vi "Open App Help file.vi"(7 "Help Tag (\"\")":string, 11 "error In":errorcluster, 13 "file name(\"App\".chm)":string) -> (15 "error out":errorcluster)   [LabVIEW 2011]
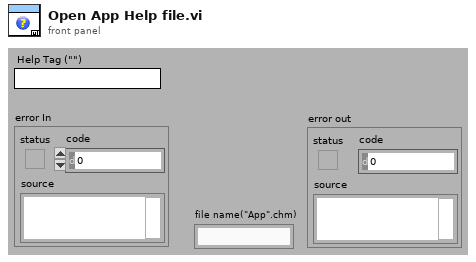
[diagram p1: front panel]
types:
  T1 = typedef "emi_Version Info.ctl" = cluster{"Name":string, "Major":i16, "Minor":i16, "Fix":i16, "Build":i32, "Type":enum16{"Alfa", "Beta", "Stable"}, "Dev":bool, "Version Name":string, "Date":timestamp}
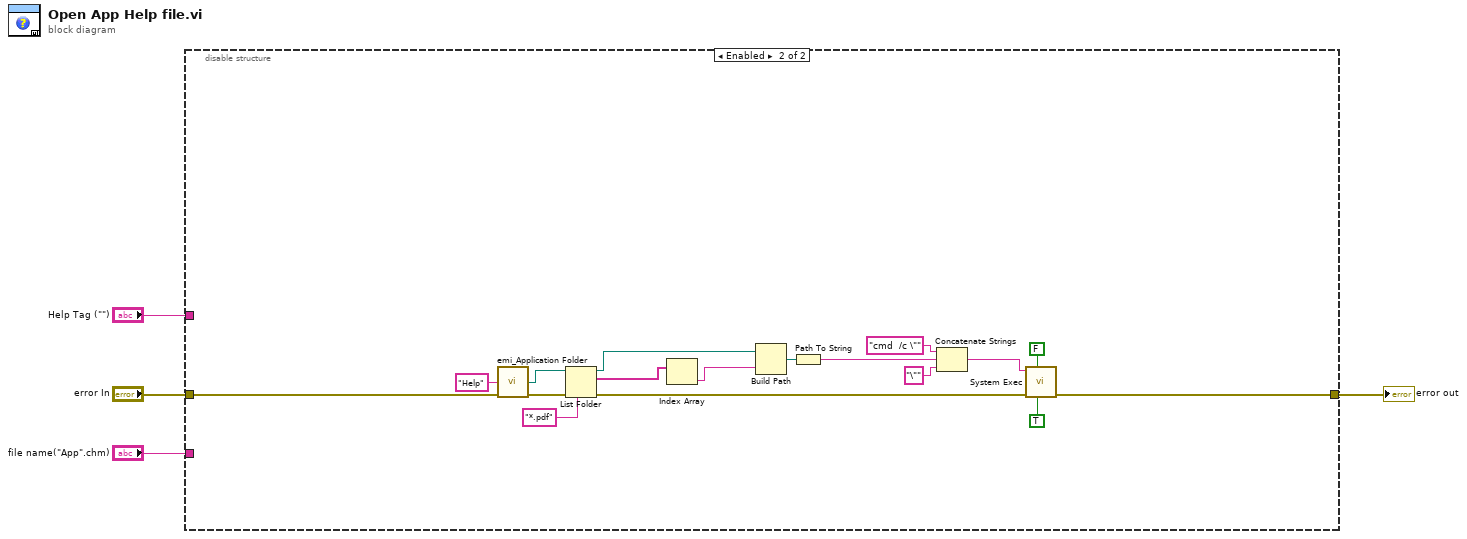
[diagram p0: block diagram]
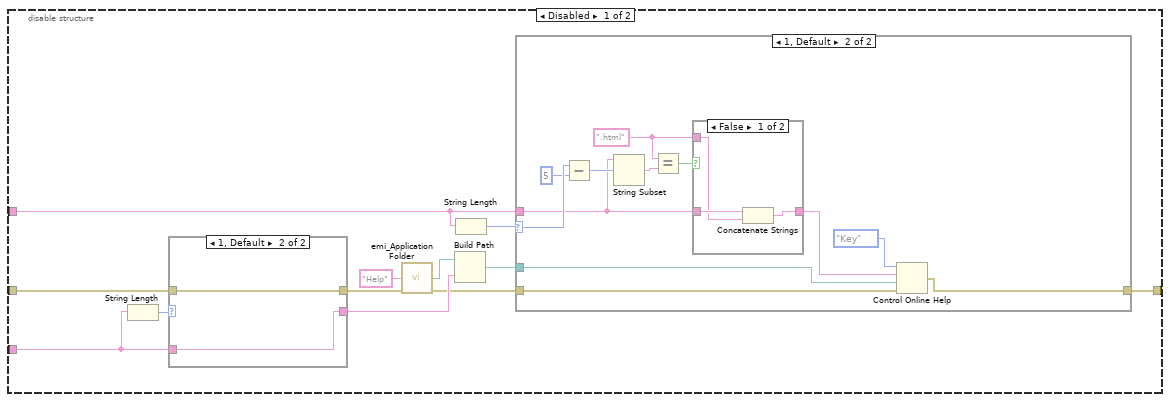
[diagram p2: hidden frame]
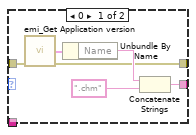
[diagram p3: hidden frame]
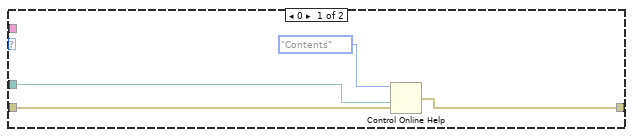
[diagram p4: hidden frame]
diagram:
  n1 = disable-structure shown="Enabled" {
    disable-tunnel: "Help Tag (\"\")" -> [w15 _]
    disable-tunnel: "error In" -> [w10 w60]
    disable-tunnel: [w7 w54] -> w2
    disable-tunnel: "file name(\"App\".chm)" -> [w5 _]
    frame Disabled {
      n2 = String Length(string=w5) -> (length=w6:i32)
      n3 = case shown="1, Default" w6 {
        tunnel: [w20 w23] -> w14
        tunnel: [w18 w24] -> w13
        tunnel: w10 -> [w17 w24]
        tunnel: w5 -> [_ w23]
        frame 0 {
          n4 = call "emi_Get Application version.vi"("error in (no error)"=w17) -> ("Version Info out"=w19:T1, "error out"=w18:errorcluster)  [unwired: 12 in, 1 out]
          n5 = Unbundle By Name(w19) -> ("Name"=w22:string)
          n6 = Concatenate Strings(w22, ".chm" ("name or relative path")) -> (w20:string)
        }
        frame 1, Default {
        }
      }
      n7 = call "emi_Application Folder.vi"("Sub Dir name"="Help", "error in (no error)"=w13) -> ("Dir"=w8:path, "error out"=w11:errorcluster)  [unwired: 12 in]
      n8 = Build Path(base path=w8, name or relative path=w14) -> (appended path=w12:path)
      n9 = String Length(string=w15) -> (length=w16:i32)
      n10 = case shown="1, Default" w16 {
        selector: w16 -> [_ w36]
        tunnel: w11 -> [w26 w40]
        tunnel: [w28 w39] -> w7
        tunnel: w15 -> [_ w31]
        tunnel: w12 -> [w25 w37]
        frame 0 {
          n11 = Control Online Help(1:w26, 2:w25, 4:enum16{"Contents", "Key", "Close"}."Contents" ("Operation")) -> (0:w28:errorcluster)  [unwired: 1 in]
        }
        frame 1, Default {
          w29 = ".html" ("x")
          n12 = Subtract(x=w36, y=5) -> (x-y=w34:i32)
          n13 = String Subset(string=w31, offset (0)=w34) -> (substring=w33:string)  [unwired: 1 in]
          n14 = Equal?(x=w29, y=w33) -> (x = y?=w32:bool)
          n15 = case shown="False" w32 {
            tunnel: w31 -> [w42 w44]
            tunnel: [w43 w44] -> w30
            tunnel: w29 -> [w41 _]
            frame False {
              n16 = Concatenate Strings(w42, w41) -> (w43:string)
            }
            frame True {
            }
          }
          n17 = Control Online Help(1:w40, 2:w37, 3:w30, 4:enum16{"Contents", "Key", "Close"}."Key" ("Operation")) -> (0:w39:errorcluster)
        }
      }
    }
    frame Enabled {
      n18 = call "emi_Application Folder.vi"("Sub Dir name"="Help", "error in (no error)"=w60) -> ("Dir"=w58:path, "error out"=w59:errorcluster)  [unwired: 12 in]
      n19 = List Folder(path=w58, pattern="*.pdf", error in=w59) -> (path out=w51:path, filenames=w56:string[], error out=w55:errorcluster)  [unwired: 1 in, 1 out]
      n20 = Index Array(array=w56) -> (element=w50:string)  [unwired: 1 in]
      n21 = Build Path(base path=w51, name or relative path=w50) -> (appended path=w49:path)
      n22 = Path To String(path=w49) -> (string=w48:string)
      n23 = Concatenate Strings("cmd  /c \"", w48, "\"") -> (w47:string)
      n24 = call <vilib>:"System Exec.vi"("run minimized? (F)"=TRUE, "wait until completion? (T)"=FALSE, "error in (no error)"=w55, "command line"=w47) -> ("error out"=w54:errorcluster)  [unwired: 4 in, 3 out]
    }
  }
  "error out" <- w2
